vi "Perform Step.vi"(8 "error in (no error)":errorcluster, 11 "Visible Assertion in":refnum<class "Visible Assertion.lvclass">) -> (0 "error out":errorcluster, 2 "Result":T1, 3 "Visible Assertion out":refnum<class "Visible Assertion.lvclass">)   [LabVIEW 2020, in "MacroAssert.lvlib" / "Visible Assertion.lvclass"]
uses:
  Visible Assertion.lvclass
  Visible Assertion.lvclass/Visible Assertion.ctl
  MacroAssert.lvlib
  CTLs/Report Data.ctl
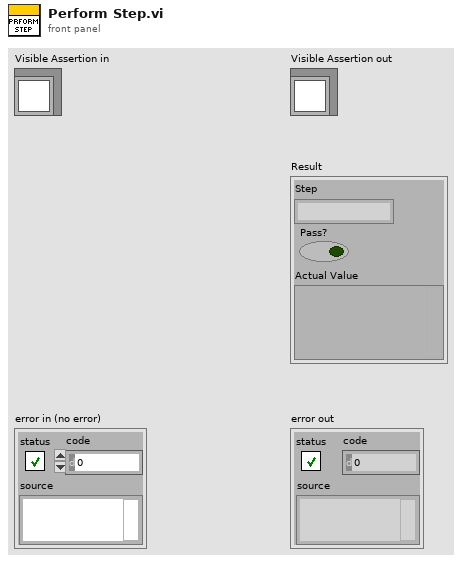
[diagram p1: front panel]
types:
  T1 = typedef "MacroAssert.lvlib/Report Data.ctl" = cluster{"Step":string, "Pass?":bool, "Actual Value":variant}
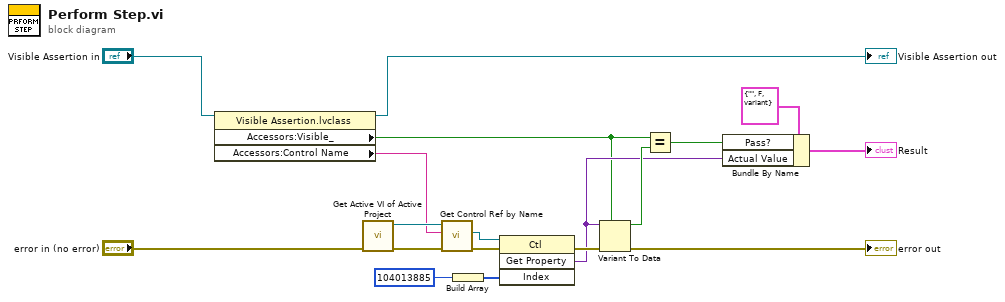
[diagram p0: block diagram]
diagram:
  n1 = property class="Visible Assertion.lvclass"(reference="Visible Assertion in") -> (reference out=→"Visible Assertion out":refnum<class "Visible Assertion.lvclass">, "Accessors:Visible_"=w1:bool, "Accessors:Control Name"=w3:string)  [unwired: 1 in, 1 out]
  n2 = call "Get Active VI of Active Project.vi"("error in (no error)"="error in (no error)") -> ("error out"=w18:errorcluster, "Active VI Ref"=w17:refnum<vi>)  [unwired: 9 in]
  n3 = call "Get Control Ref by Name.vi"("error in (no error)"=w18, "Name"=w3, "VI Ref"=w17) -> ("error out"=w15:errorcluster, "Ctl Ref"=w11:refnum<vi>)  [unwired: 6 in, 1 out]
  n4 = Build Array(104013885) -> (w13:i32[])
  n5 = invoke class="Ctl" method="Get Property"(reference=w11, error in=w15, "Index"=w13) -> (error out=w16:errorcluster, "GetProperty"=w9:variant)  [unwired: 1 in, 2 out]
  n6 = Variant To Data(error in=w16, type=w1, Variant=w9) -> (data=w12:bool, error out=→"error out":errorcluster)
  n7 = Equal?(x=w1, y=w12) -> (x = y?=w10:bool)
  n8 = Bundle By Name(cluster=T1 {"Step"="", "Pass?"=FALSE, "Actual Value"=variant} ("Report Data"), "Pass?"=w10, "Actual Value"=w9) -> (→"Result":T1)
